vi "DAQ-Data-to-File Settings Dialog.vi"(8 "error in (no error)":errorcluster, 11 "Configuration in":T1={"Hardware Configuration"={"HW Refnum <Replace Me>"="", "Signal Type <Replace Me>"=enum."Sine Wave"}, "Analysis Configuration"={"Statistics"=TRUE}, "New Data Behavior"=enum."Replace"}) -> (0 "error out":errorcluster, 2 "UI Refresh Needed?":bool, 3 "Configuration out":T1={"Hardware Configuration"={"HW Refnum <Replace Me>"="", "Signal Type <Replace Me>"=enum."Sine Wave"}, "Analysis Configuration"={"Statistics"=TRUE}, "New Data Behavior"=enum."Replace"})   [LabVIEW 2020]
doc: "Dialog for selecting user specified settings."
uses:
  controls/DAQ-Data-to-File User Specified Data.ctl
  controls/DAQ-Data-to-File HW Configuration.ctl
  controls/DAQ-Data-to-File Simulated Signal Type.ctl
  controls/DAQ-Data-to-File Analysis Configuration.ctl
  controls/DAQ-Data-to-File New Data Behavior.ctl
panel:
  in  "Signal Type":u16(ring) items=["Sine Wave", "Square Wave"]
  in  "New Data Behavior":u16(ring) items=["Replace", "Overlay", "Append"]
  in  "Cancel Button":bool
  in  "OK Button":bool
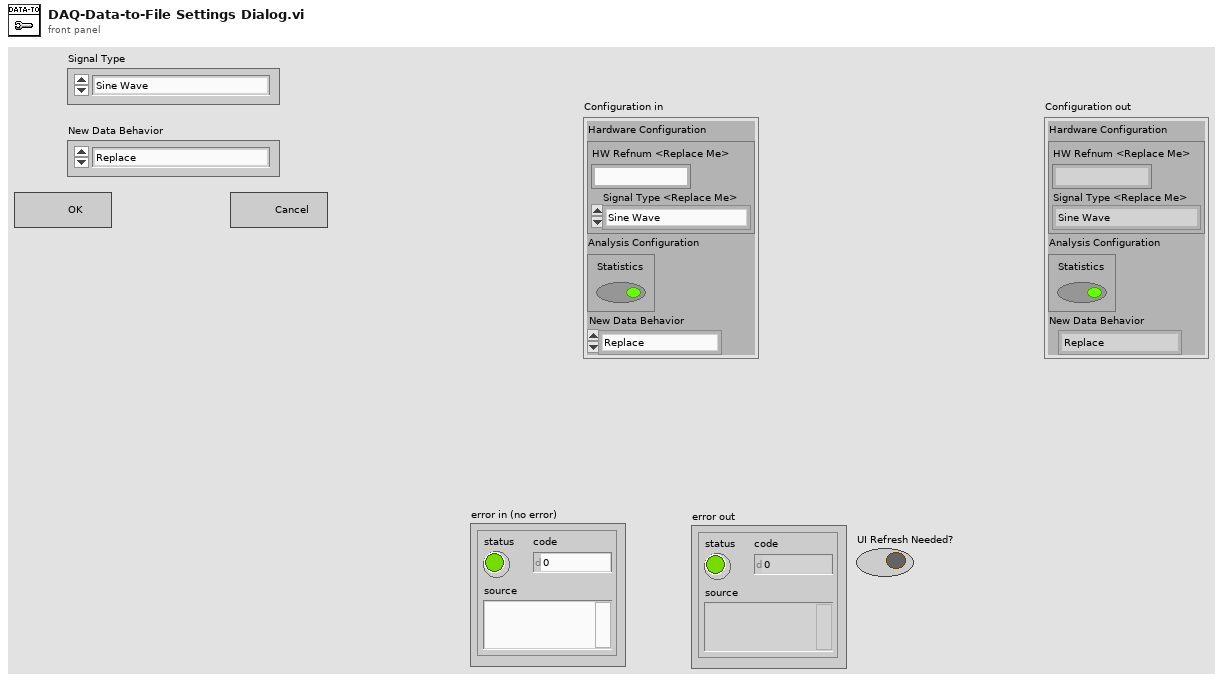
[diagram p1: front panel]
types:
  T1 = typedef "DAQ-Data-to-File User Specified Data.ctl" = cluster{"Hardware Configuration":T2, "Analysis Configuration":T4, "New Data Behavior":T5}
  T2 = typedef "DAQ-Data-to-File HW Configuration.ctl" = cluster{"HW Refnum <Replace Me>":string, "Signal Type <Replace Me>":T3}
  T3 = typedef "DAQ-Data-to-File Simulated Signal Type.ctl" = enum16{"Sine Wave", "Square Wave"}
  T4 = typedef "DAQ-Data-to-File Analysis Configuration.ctl" = cluster{"Statistics":bool}
  T5 = typedef "DAQ-Data-to-File New Data Behavior.ctl" = enum16{"Replace", "Overlay", "Append"}
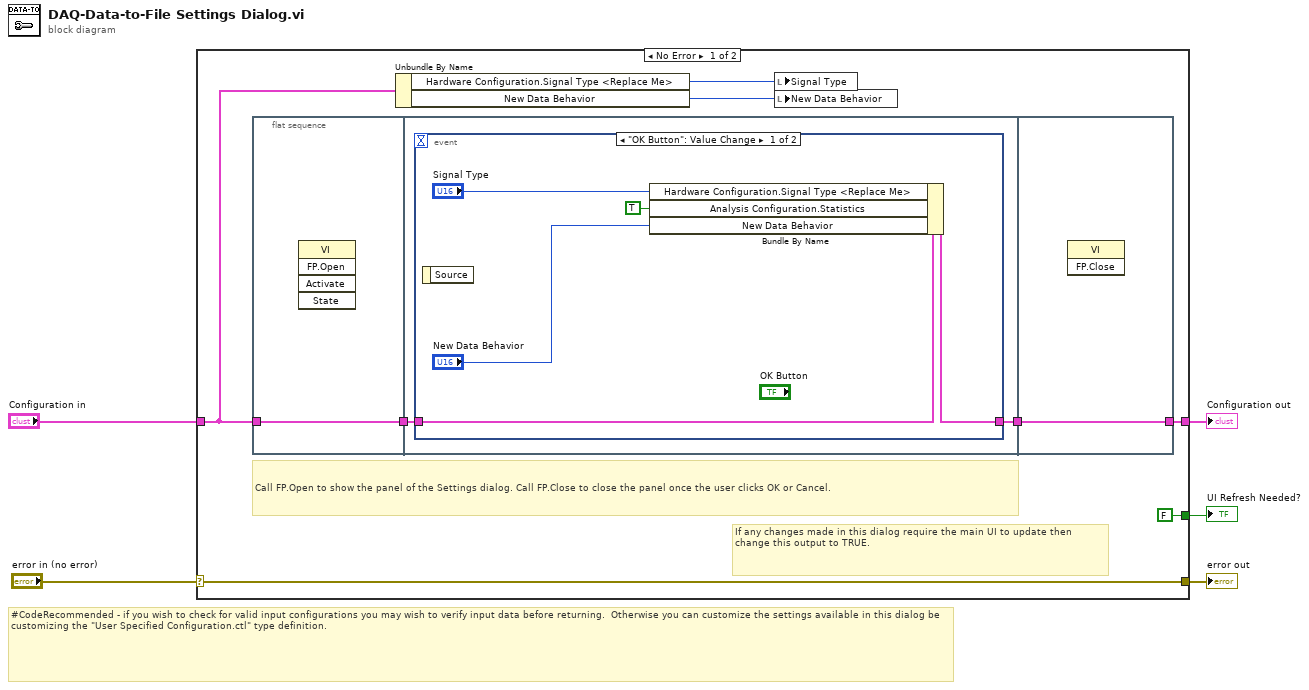
[diagram p0: block diagram]
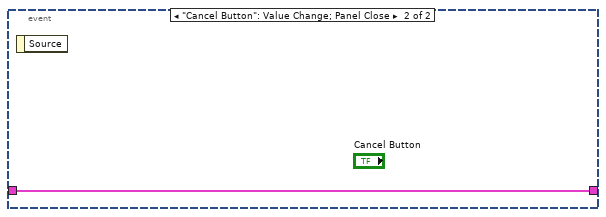
[diagram p2: hidden frame]
diagram:
  # "#CodeRecommended - if you wish to check for valid input configurations you may wish to verify input data before returning.  Otherwise you can customize the settings available in this dialog be customizing the \"User Specified Configuration.ctl\" type definition."
  n1 = case shown="No Error" "error in (no error)" {
    selector: "error in (no error)" -> [w13 w25]
    tunnel: [w13 w25] -> w4
    tunnel: "Configuration in" -> [w10 w24]
    tunnel: [w12 w24] -> w2
    tunnel: [FALSE ("UI Refresh Needed?") _] -> w1
    frame No Error {
      # "Call FP.Open to show the panel of the Settings dialog. Call FP.Close to close the panel once the user clicks OK or Cancel."
      # "If any changes made in this dialog require the main UI to update then change this output to TRUE."
      n2 = flat-sequence {
        tunnel: w10 -> [w14]
        tunnel: [w14] -> w7
        tunnel: w7 -> [w15]
        tunnel: [w16] -> w6
        tunnel: [w23] -> w12
        tunnel: w6 -> [w23]
        frame #0 {
          n3 = invoke class="VI" method="FP.Open"() -> ()  [unwired: 5 in, 5 out]
        }
        frame #1 {
          n4 = event shown="[0] \"OK Button\": Value Change" {
            selector: _ -> [_ _]
            dyn-events: _ -> [_ _]
            timeout: _ -> [_ _]
            tunnel: [w20 w22] -> w16
            tunnel: w15 -> [w21 w22]
            event "OK Button": Value Change {
              n5 = event-data() -> ()  [unwired: 1 in, 1 out]
              n6 = Bundle By Name(cluster=w21, "Hardware Configuration.Signal Type <Replace Me>"="Signal Type", "Analysis Configuration.Statistics"=TRUE, "New Data Behavior"="New Data Behavior") -> (w20:T1)
            }
            event "Cancel Button": Value Change; Panel Close {
              n7 = event-data() -> ()  [unwired: 1 in, 1 out]
            }
          }
        }
        frame #2 {
          n8 = invoke class="VI" method="FP.Close"() -> ()  [unwired: 3 in, 3 out]
        }
      }
      n9 = Unbundle By Name(w10) -> ("Hardware Configuration.Signal Type <Replace Me>"=w9:T3, "New Data Behavior"=w8:T5)
      n10 = local write "Signal Type"(w9) -> ()
      n11 = local write "New Data Behavior"(w8) -> ()
    }
    frame Error {
    }
  }
  "UI Refresh Needed?" <- w1
  "error out" <- w4
  "Configuration out" <- w2
